vi "Strings.vi"(8 "Array 2":T1(array[cluster])=[{"String"="Dallas", "Combo Box"="North of Austin", "Path"=path "C:/Program Files/National Instruments/TestStand 4.2/Bin/SeqEdit.exe", "Cluster"={"Array"=["AAAaaa", "HHhh", "DDdd", "abcdhd"]}}, {"String"="Richardson", "Combo Box"="Dallas City", "Path"=path "\\\\nirvana\\temp/jah/DefaultValues/7.1.1/New Set/EnumControl.ctl", "Cluster"={"Array"=["AAA", "HHHH", "DDDDDD"]}}], 9 "Array":string[](array[string])=["ABC", "DEF", "GHIJ"], 10 "Cluster":T2={"String"="Austin", "Combo Box"="Austin City", "Path"=path "\\\\nirvana\\temp/jah/DefaultValues/7.1.1/New Set/Strings.vi", "Cluster"={"Array"=["AAA", "HHHH", "DDDDDD"]}}, 11 "String":string="Texas") -> ()   [LabVIEW 2011]
panel:
  in  "stop":bool
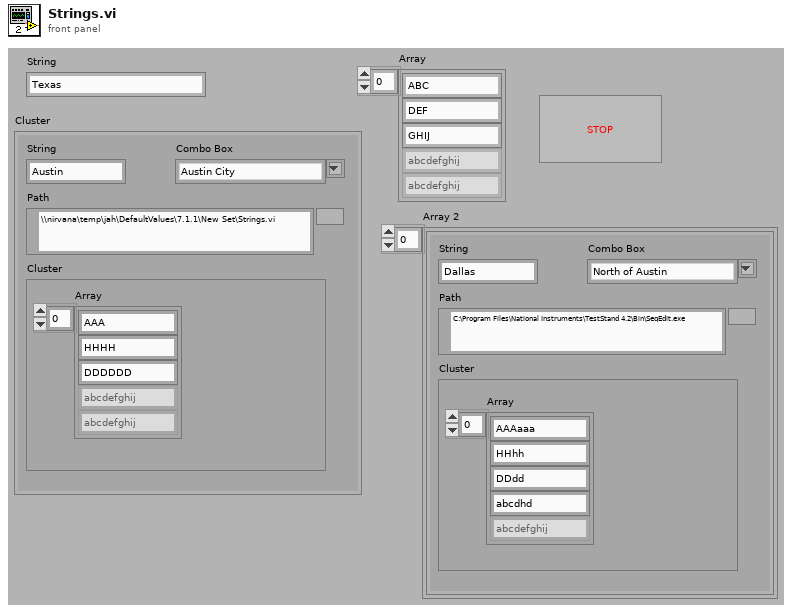
[diagram p1: front panel]
types:
  T1 = cluster{"String":string, "Combo Box":string, "Path":path, "Cluster":cluster{"Array":string[]}}[]
  T2 = cluster{"String":string, "Combo Box":string, "Path":path, "Cluster":cluster{"Array":string[]}}
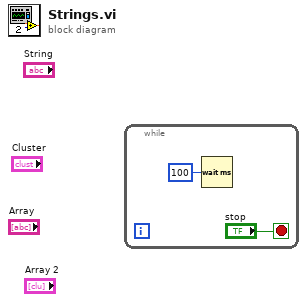
[diagram p0: block diagram]
diagram:
  n1 = while {
    stop <- "stop" stop-if-true
    n2 = Wait (ms)(milliseconds to wait=u32 100) -> ()  [unwired: 1 out]
  }
